vi "trivial.vi"(11 "IN":dbl) -> (0 "OUT":dbl)   [LabVIEW 2009]
panel:
  in  "stop":bool
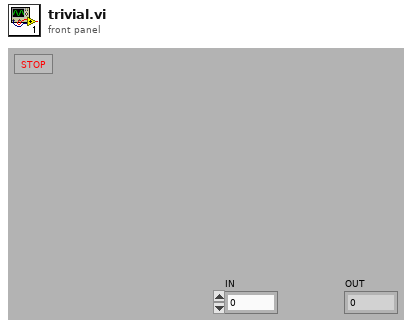
[diagram p1: front panel]
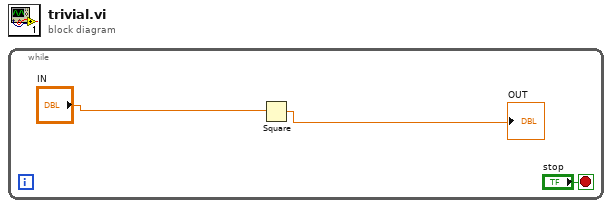
[diagram p0: block diagram]
diagram:
  n1 = while {
    stop <- "stop" stop-if-true
    n2 = Square(x="IN") -> (x^2=→"OUT":dbl)
  }
